vi "POST-Multipart.vi"(6 "timeout":i32=10000, 7 "output file":path, 8 "error in":errorcluster, 9 "Multipart Post data":T1[](array[typedef]), 10 "url":string, 11 "http-client in":refnum<class "http-client.lvclass">) -> (0 "error out":errorcluster, 1 "body":string, 2 "headers":string, 3 "http-client out":refnum<class "http-client.lvclass">)   [LabVIEW 2020, in "REST Client.lvlib" / "http-client.lvclass"]
uses:
  http-client.lvclass
  <vilib>/httpClient/MultipartData.ctl
  <vilib>/httpClient/LabVIEWHTTPClient.lvlib
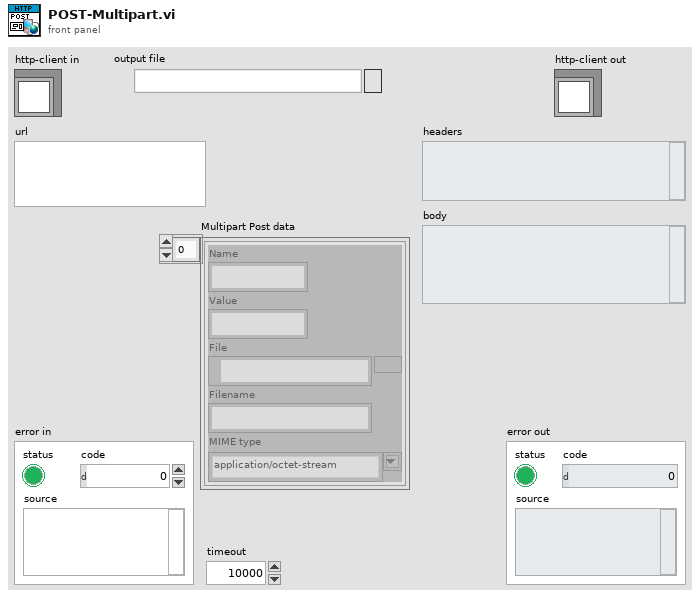
[diagram p1: front panel]
types:
  T1 = typedef "LabVIEWHTTPClient.lvlib/MultipartData.ctl" = cluster{"Name":string, "Value":string, "File":path, "Filename":string, "MIME type":string}
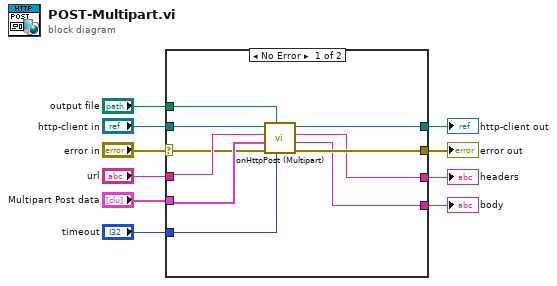
[diagram p0: block diagram]
diagram:
  n1 = case shown="No Error" "error in" {
    selector: "error in" -> [w16 w22]
    tunnel: [w15 w22] -> w9
    tunnel: [w14 w21] -> w7
    tunnel: "http-client in" -> [w20 w21]
    tunnel: [w12 _] -> w6
    tunnel: "url" -> [w17 _]
    tunnel: "timeout" -> [w19 _]
    tunnel: "output file" -> [w13 _]
    tunnel: [w11 _] -> w2
    tunnel: "Multipart Post data" -> [w18 _]
    frame No Error {
      n2 = call-dynamic "onHttpPost (Multipart).vi"("timeout"=w19, "output file"=w13, "error in"=w16, "Multipart Post data"=w18, "url"=w17, "http-method in"=w20) -> ("error out"=w15:errorcluster, "body"=w11:string, "headers"=w12:string, "http-method out"=w14:refnum<class "http-client.lvclass">)  [unwired: 2 in]
    }
    frame Error {
    }
  }
  "error out" <- w9
  "http-client out" <- w7
  "headers" <- w6
  "body" <- w2
